vi "Configure Trigger Delay.vi"(8 "error in (no error)":errorcluster, 9 "Delay Time (2.00E-008)":dbl=2e-08 format="%.2e", 11 "VISA resource name":refnum<visa-resource-name>) -> (0 "error out":errorcluster, 3 "VISA resource name out":refnum<visa-resource-name>)   [LabVIEW 2020, in "Rohde&Schwarz RTx Oscilloscopes.lvlib"]
doc: "This VI sets the time the instrument waits after an A-event until it recognizes B-events.\n\nAttribute:\nRSRTX_ATTR_TRIGGER_DELAY\n\nRemote-control command:\nTRIGger:B:DELay"
uses:
  Rohde&Schwarz RTx Oscilloscopes.lvlib
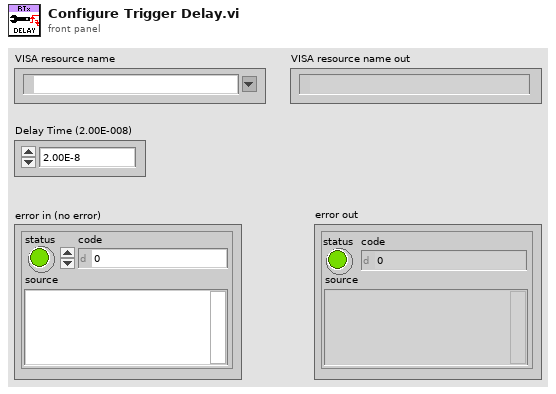
[diagram p1: front panel]
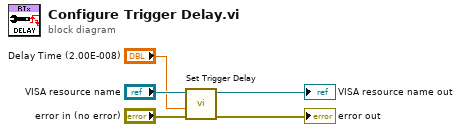
[diagram p0: block diagram]
diagram:
  n1 = call "Set Trigger Delay"("error in (no error)"="error in (no error)", "Trigger Delay (0.0)"="Delay Time (2.00E-008)", "instrument handle"="VISA resource name") -> ("error out"=→"error out":errorcluster, "instrument handle out"=→"VISA resource name out":refnum<visa-resource-name>)  [unwired: 7 in]
